vi "Update Digital Multiple.vi"(8 "error in (no error)":errorcluster, 10 "Channels":T1[](array[typedef]), 11 "SoftVar Module in":refnum<class "SoftVar Module.lvclass">) -> (0 "error out":errorcluster, 3 "SoftVar Module out":refnum<class "SoftVar Module.lvclass">)   [LabVIEW 2020, in "Volatus.lvlib" / "SoftVar Module.lvclass"]
uses:
  SoftVar Module.lvclass
  SoftVar Module.lvclass/SoftVar Module.ctl
  Batch Update.ctl
  <vilib>/Utility/miscctls.llb/LVMapReplaceAction.ctl
  lv-vecto/Vecto/Group DBL/Group DBL.lvclass
  VolatusAPI/VolatusAPI.lvclass
  Module/Module.lvclass
  C:/dev/lv20CE/relink/lv-volatus/Volatus/Module/Module.lvclass
  C:/dev/lv20CE/relink/lv-volatus/Volatus/SoftVar Module/SoftVar Module.lvclass
  lv-vecto/Vecto/Vecto.lvlib
  messages/CmdDigital/Data.ctl
  messages/CmdDigital/CmdDigital.lvlib
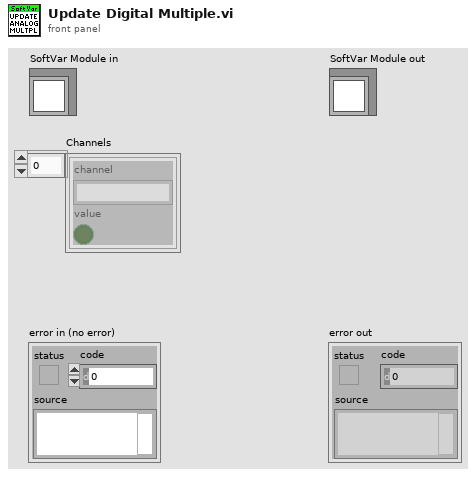
[diagram p1: front panel]
types:
  T1 = typedef "CmdDigital.lvlib/Data.ctl" = cluster{"channel":string, "value":bool}
  T2 = typedef "LVMapReplaceAction.ctl" = enum32{"Modify Entry only if found", "Add or Modify Entry", "Delete Entry"}
  T3 = typedef "Volatus.lvlib/SoftVar Module.lvclass/Batch Update.ctl" = cluster{"Indices":i32[], "Values":dbl[]}
  T4 = typedef "Volatus.lvlib/SoftVar Module.lvclass/Channel Info.ctl" = cluster{"Group Index":i32, "Index":i32}
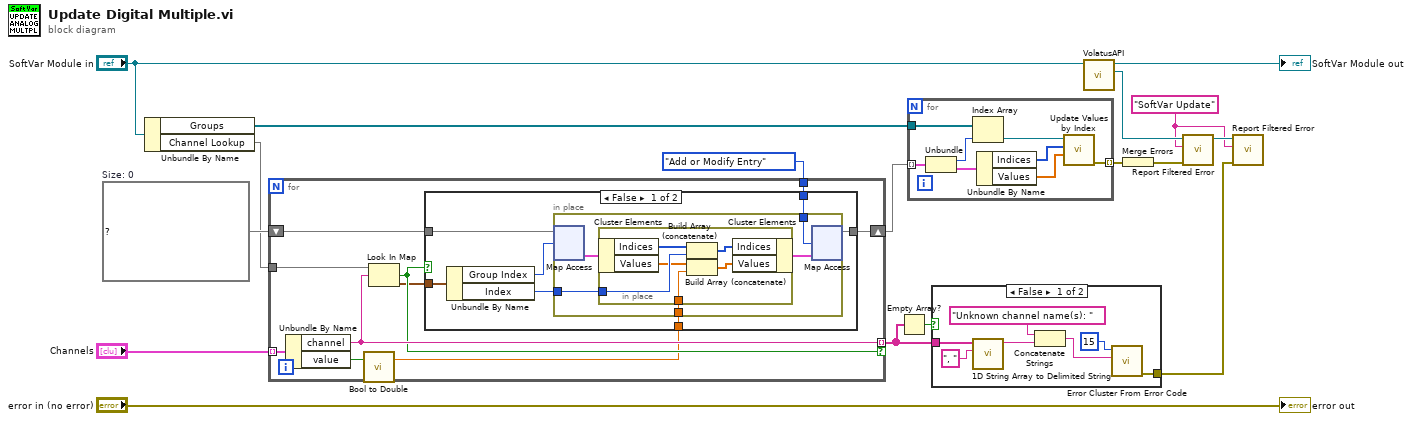
[diagram p0: block diagram]
diagram:
  w2 = "SoftVar Update" ("Context")
  w15 = map{i32, T3} {}  # Size: 0
  n1 = Unbundle By Name("SoftVar Module in") -> ("Groups"=w11:refnum<class "Group DBL.lvclass">[], "Channel Lookup"=w14:map{string, T4})
  n2 = for {
    tunnel: "Channels" -> [w27] mode=indexing
    shift-right: [w21] -> w12
    shift-left: w15 -> [w22]
    tunnel: w14 -> [w26]
    tunnel: [w25] -> w8 mode=indexing if=w24
    tunnel: LVMapReplaceAction."Add or Modify Entry" ("action") -> [w19]
    n3 = Unbundle By Name(w27) -> ("channel"=w25:string, "value"=w20:bool)
    n4 = call "Bool to Double.vi"("Bool"=w20) -> ("Double"=w18:dbl)  [unwired: 2 in]
    n5 = Look In Map(map=w26, key=w25) -> (key not found?=w24:bool, value=w23:T4)  [unwired: 1 in]
    n6 = case shown="False" w24 {
      tunnel: w23 -> [w34 _]
      tunnel: w22 -> [w33 w46]
      tunnel: [w29 w46] -> w21
      tunnel: w18 -> [w30 _]
      tunnel: w19 -> [w28 _]
      frame False {
        n7 = Unbundle By Name(w34) -> ("Group Index"=w32:i32, "Index"=w31:i32)
        n8 = in-place {
          in-place-border: w31 -> [w38]
          in-place-border: w30 -> [w37]
          in-place-border: w28 -> [w35]
          n9 = in-place-map #1(w33, w32) -> (w39:T3)  [unwired: 1 in, 1 out]
          n10 = in-place {
            in-place-border: w38 -> [w44]
            in-place-border: w37 -> [w40]
            n11 = in-place-cluster #2(w39) -> ("Indices"=w45:i32[], "Values"=w43:dbl[])
            n12 = Build Array (concatenate)(w45, w44) -> (w41:i32[])
            n13 = Build Array (concatenate)(w43, w40) -> (w42:dbl[])
            n14 = in-place-cluster #2("Indices"=w41, "Values"=w42) -> (w36:T3)
          }
          n15 = in-place-map #1(w36, w35) -> (w29:map{i32, T3})  [unwired: 2 out]
        }
      }
      frame True {
      }
    }
  }
  n16 = Empty Array?(array=w8) -> (empty?=w9:bool)
  n17 = for {
    tunnel: w12 -> [w54] mode=indexing
    tunnel: w11 -> [w53]
    tunnel: [w47] -> w10 mode=indexing
    n18 = Unbundle(w54) -> ("Group Index"=w52:i32, "Batch Update"=w51:T3)
    n19 = Index Array(array=w53, index=w52) -> (element=w50:refnum<class "Group DBL.lvclass">)
    n20 = Unbundle By Name(w51) -> ("Indices"=w49:i32[], "Values"=w48:dbl[])
    n21 = call "Update Values by Index.vi"("Scaled"=w48, "Index"=w49, "Group in"=w50) -> ("error out"=w47:errorcluster)  [unwired: 7 in, 1 out]
  }
  n22 = case shown="False" w9 {
    tunnel: w8 -> [w61 _]
    tunnel: [w55 _] -> w1
    frame False {
      n23 = call <vilib>:"1D String Array to Delimited String.vi"("delimiter"=", ", "string array"=w61) -> ("delimited string"=w58:string)  [unwired: 9 in]
      n24 = Concatenate Strings("Unknown channel name(s): ", w58) -> (w56:string)
      n25 = call <vilib>:"Error Cluster From Error Code.vi"("error message (\"\")"=w56, "error code (0)"=15) -> ("error out"=w55:errorcluster)  [unwired: 7 in]
    }
    frame True {
    }
  }
  n26 = call "VolatusAPI.vi"("Module in"="SoftVar Module in") -> ("VolatusAPI"=w4:refnum<class "VolatusAPI.lvclass">, "Module out"=→"SoftVar Module out":refnum<class "SoftVar Module.lvclass">)  [unwired: 9 in]
  n27 = Merge Errors(w10) -> (w7:errorcluster)
  n28 = call "Report Filtered Error.vi"("error in (no error)"=w7, "Context"=w2, "VolatusAPI in"=w4) -> ("VolatusAPI out"=w3:refnum<class "VolatusAPI.lvclass">)  [unwired: 7 in, 1 out]
  n29 = call "Report Filtered Error.vi"("error in (no error)"=w1, "Context"=w2, "VolatusAPI in"=w3) -> ()  [unwired: 7 in, 2 out]
  "error out" <- "error in (no error)"
